vi "part2.vi"() -> ()   [LabVIEW 2018]
panel:
  in  "stop":bool
  out "selector":dbl
  out "equal":bool
  out "less":bool
  out "greater":bool
  in  "selector switch":bool
  in  "input b":dbl
  in  "input a":dbl
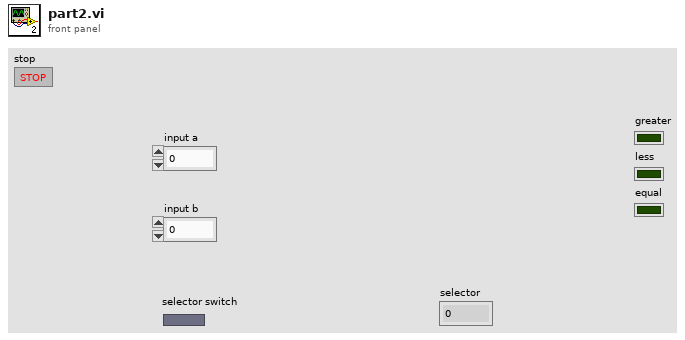
[diagram p1: front panel]
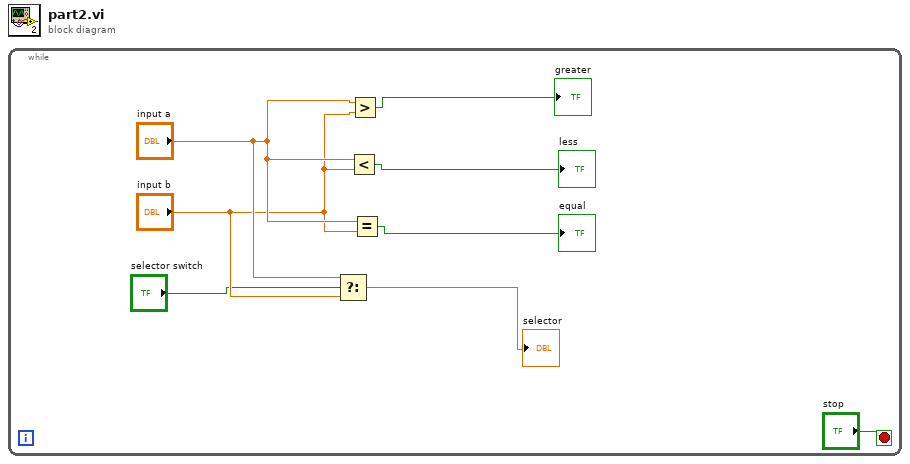
[diagram p0: block diagram]
diagram:
  n1 = while {
    stop <- "stop" stop-if-true
    n2 = Select(t="input a", s="selector switch", f="input b") -> (s? t:f=→"selector":dbl)
    n3 = Less?(x="input a", y="input b") -> (x < y?=→"less":bool)
    n4 = Greater?(x="input a", y="input b") -> (0:→"greater":bool)
    n5 = Equal?(x="input a", y="input b") -> (x = y?=→"equal":bool)
  }
